vi "prepAI_ttv2.vi"(2 "triggersource":tag) -> (0 "Terminal Name with Device Prefix":tag)   [LabVIEW 2015]
uses:
  <vilib>/DAQmx/create/channels.llb/DAQmx Create Channel (AI-Voltage-Basic).vi
  <vilib>/DAQmx/configure/timing.llb/DAQmx Timing (Sample Clock).vi
  <vilib>/DAQmx/configure/trigger.llb/DAQmx Start Trigger (Digital Edge).vi
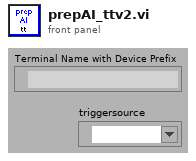
[diagram p1: front panel]
types:
  T1 = cluster{"StageS":i32, "StageL":i32, "currmeas data dir":path, "image OD":u16, "contour OD":u16, "point OD":u16, "AOlines":tag[], "AIlines":tag[], "CI lines":tag[], "DO lines":tag[], "AO names":string[], "CI names":string[], "AI names":string[], "DO names":string[], "CIextensions":string[], "AIextensions":string[], "Voltage to Ygalvo":i32, "Voltage to Xgalvo":i32, "Voltage to patch":i32, "640 shutter":i32, "2P shutter":i32, "LT timestamp":u32, "Vp":i32, "Ip":i32, "camera trigger":i32, "master data dir":path, "voltage to Zpos":i32, "Vto2P":i32, "640 AO":i32, "488 AO":i32, "532 AO":i32, "640TTL":u32, "488TTL":u32, "532TTL":u32, "Device 1 sampleclock out":tag, "Device 1 Starttrigger out":tag, "Device 2 sampleclock in":tag, "Device 2 StartTrigger in ":tag, "2PODTTL":u32, "488 shutter":u32, "LCVR red":u32, "LCVR blue":u32}
  T2 = typedef "LVRectTypeDef.ctl" = cluster{"Left":i16, "Top":i16, "Right":i16, "Bottom":i16}
  T3 = cluster{"Xpixels":i32, "Vxminref":dbl, "Vxmaxref":dbl, "P":dbl, "Ypixels":i32, "Vyminref":dbl, "Vymaxref":dbl, "srate":sgl, "sAOxy":i32, "timeout":dbl, "type":string, "date":string, "time":string, "Colormap":u16, "Drawing Mode":u16, "Scanning Mode":u16, "square pixels":bool, "square matrix":bool, "Xpixels Img":i32, "Vx-min Img":dbl, "VX-max Img":dbl, "Ypixels Img":i32, "Vy-min Img":dbl, "Vy-max Img ":dbl, "Angle Img":dbl, "autoshutter":bool, "finite":bool, "cont":bool, "wavdet":bool, "measpoints":i32, "avpp":i32, "bufferAO":i32, "bufferAI":i32, "starttick":u32, "waveform":path, "Vx-ref":dbl, "Vy-ref":dbl, "refreshrate":dbl, "refreshbuffer":i32, "tt_cycles":i32, "motorref":refnum<k7>, "mirrorswitch":refnum<k7>, "sample mode":i32, "maxbufferAI":i32, "srateAODO":sgl, "bin":sgl, "Pel":sgl, "Angle draw":dbl, "srate Img":sgl, "ROIimg_plotbounds":T2, "auto OD":bool, "ODfilt":u16, "aAI":i32[], "aCI":i32[], "aAO":u32[], "aDO":u32[], "refwfsize":dbl, "Lifetime":bool, "Vz-Img":dbl, "Vz-ref":dbl, "Vz-reset":dbl, "AIoverride":bool}
  T4 = cluster{" AI":refnum<k21>, "E_AI":errorcluster, "header":dbl[]}
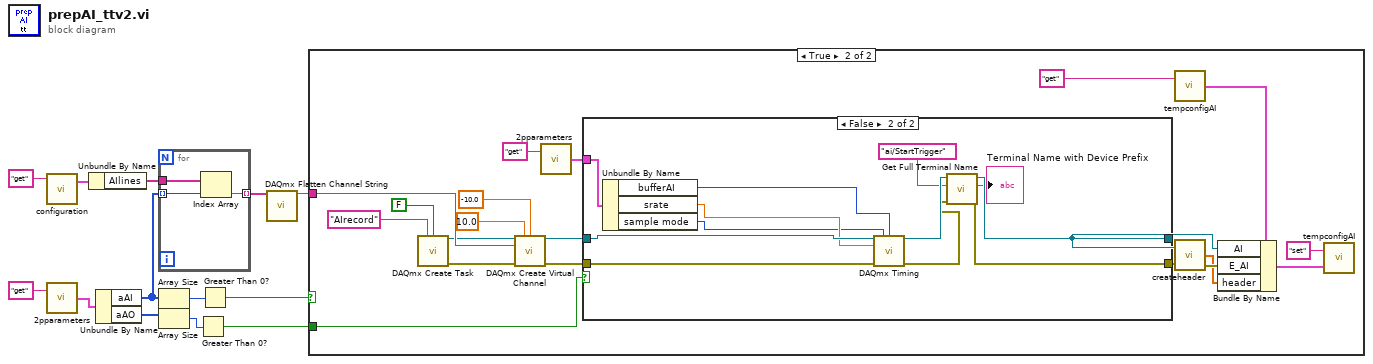
[diagram p0: block diagram]
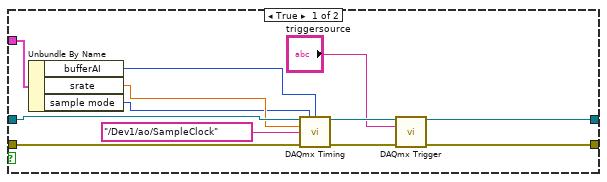
[diagram p3: hidden frame]
diagram:
  n1 = call "configuration.vi"("command"="get") -> ("config out"=w10:T1)  [unwired: 2 in, 1 out]
  n2 = call "2pparameters.vi"("command"="get") -> ("params out"=w11:T3)  [unwired: 1 in]
  n3 = Unbundle By Name(w10) -> ("AIlines"=w9:tag[])
  n4 = Unbundle By Name(w11) -> ("aAI"=w4:i32[], "aAO"=w3:u32[])
  n5 = for {
    tunnel: w4 -> [w16] mode=indexing
    tunnel: w9 -> [w15]
    tunnel: [w14] -> w8 mode=indexing
    n6 = Index Array(array=w15, index=w16) -> (element=w14:tag)
  }
  n7 = Array Size(array=w4) -> (size(s)=w7:i32)
  n8 = Array Size(array=w3) -> (size(s)=w2:i32)
  n9 = Greater Than 0?(x=w2) -> (x > 0?=w1:bool)
  n10 = Greater Than 0?(x=w7) -> (x > 0?=w5:bool)
  n11 = call <vilib>:"DAQmx Flatten Channel String.vi"("names in"=w8) -> ("names out"=w6:string)  [unwired: 13 in, 1 out]
  n12 = case shown="True" w5 {
    tunnel: w6 -> [_ w32]
    tunnel: w1 -> [_ w17]
    frame False {
    }
    frame True {
      n13 = call <vilib>:"DAQmx Create Task.vi"("new task name"="AIrecord", "auto cleanup"=FALSE) -> ("task out"=w21:refnum<k21>, "error out"=w22:errorcluster)  [unwired: 12 in]
      n14 = call-poly <vilib>:"DAQmx Create Virtual Channel.vi"("task in"=w21, "maximum value"=10.0, "minimum value"=-10.0, "physical channels"=w32, "error in"=w22) -> ("task out"=w36:refnum<k21>, "error out"=w35:errorcluster)  [unwired: 9 in]
      n15 = call "2pparameters.vi"("command"="get") -> ("params out"=w34:T3)  [unwired: 1 in]
      n16 = case shown="False" w17 {
        tunnel: w36 -> [w48 w60]
        tunnel: w35 -> [w47 w59]
        tunnel: w34 -> [w46 w58]
        tunnel: [w41 w53] -> w19
        tunnel: [w39 w51] -> w18
        frame True {
          n17 = Unbundle By Name(w46) -> ("bufferAI"=w37:i32, "srate"=w45:sgl, "sample mode"=w43:i32)
          n18 = call-poly <vilib>:"DAQmx Timing.vi"("task/channels in"=w48, "sample mode"=w43, "samples per channel"=w37, "rate"=w45, "source"=tag "/Dev1/ao/SampleClock", "error in"=w47) -> ("task out"=w42:refnum<k21>, "error out"=w40:errorcluster)  [unwired: 8 in]
          n19 = call-poly <vilib>:"DAQmx Trigger.vi"("task/channels in"=w42, "source"="triggersource", "error in"=w40) -> ("task out"=w41:refnum<k21>, "error out"=w39:errorcluster)  [unwired: 11 in]
        }
        frame False {
          n20 = Unbundle By Name(w58) -> ("bufferAI"=w55:i32, "srate"=w57:sgl, "sample mode"=w56:i32)
          n21 = call-poly <vilib>:"DAQmx Timing.vi"("task/channels in"=w60, "sample mode"=w56, "samples per channel"=w55, "rate"=w57, "error in"=w59) -> ("task out"=w54:refnum<k21>, "error out"=w52:errorcluster)  [unwired: 9 in]
          n22 = call "Get Full Terminal Name.vi"("error in"=w52, "Local Terminal Name"="ai/StartTrigger", "task/channels in"=w54) -> ("error out"=w51:errorcluster, "Terminal Name with Device Prefix"=→"Terminal Name with Device Prefix":tag, "task out"=w53:refnum<k21>)  [unwired: 6 in]
        }
      }
      n23 = call "tempconfigAI.vi"("command"="get") -> ("Temp Config out"=w30:T4)  [unwired: 1 in]
      n24 = call "createheader.vi"("task in"=w19, "error in"=w18) -> ("Array"=w24:dbl[], "error out"=w25:errorcluster)  [unwired: 1 out]
      n25 = Bundle By Name(cluster=w30, "AI"=w19, "E_AI"=w25, "header"=w24) -> (w31:T4)
      n26 = call "tempconfigAI.vi"("Temp Config in"=w31, "command"="set") -> ()  [unwired: 1 out]
    }
  }
